vi "thermo_handmade_conver.vi"(8 "y":dbl=1000000.0, 10 "Measurement Data[1]":dbl, 11 "Measurement Data[0]":dbl) -> (3 "Result":dbl)   [LabVIEW 2011]
uses:
  <vilib>/express/express arith-compare/Formula/XNode/ExpressFormulaBlockNode.xnode
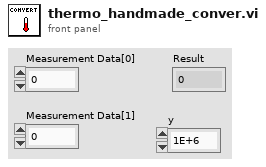
[diagram p1: front panel]
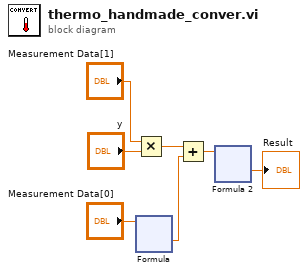
[diagram p0: block diagram]
diagram:
  n1 = Multiply(x="Measurement Data[1]", y="y") -> (x*y=w3:dbl)
  n2 = xnode ("Formula")("T"="Measurement Data[0]") -> ("Result"=w1:dbl)  [unwired: 1 in, 1 out]
  n3 = Add(x=w3, y=w1) -> (x+y=w2:dbl)
  n4 = xnode ("Formula 2")("V"=w2) -> ("Result"=→"Result":dbl)  [unwired: 1 in, 1 out]
